vi "FTW-Actor-Broker-Initialize.vi"(0 "FTW Message Broker":refnum<class "FTW-Actor-Broker.lvclass">, 5 "Initialized Response":string, 11 "error in":errorcluster) -> (4 "FTW Message Broker out":refnum<class "FTW-Actor-Broker.lvclass">, 6 "Observer":refnum<event-registration>, 15 "error out":errorcluster)   [LabVIEW 2012, in "FTW-Actor-Broker.lvclass"]
uses:
  FTW-Actor-Broker.lvclass
  Messaging/Message/FTW-Message.lvclass
  Container/FTW-Container.lvclass
panel:
  # "Inputs"
  # "Outputs"
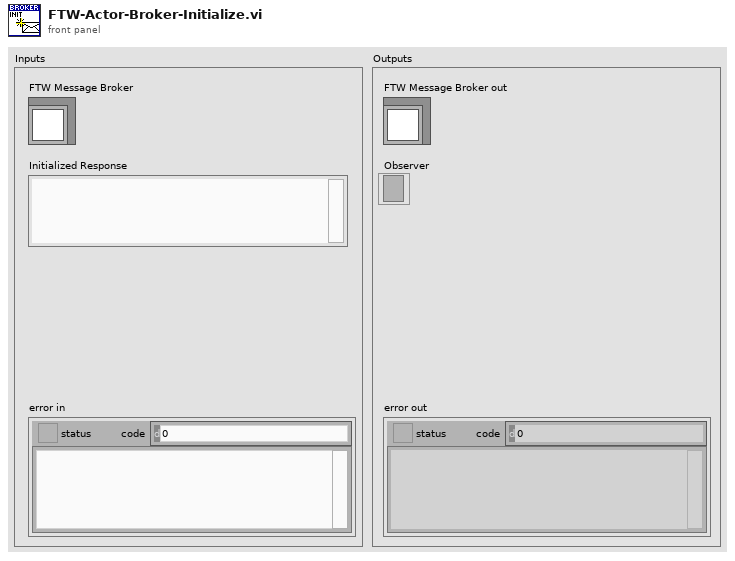
[diagram p1: front panel]
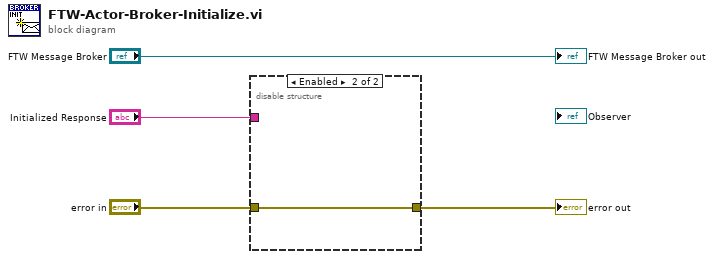
[diagram p0: block diagram]
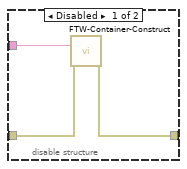
[diagram p2: hidden frame]
diagram:
  n1 = disable-structure shown="Enabled" {
    disable-tunnel: "Initialized Response" -> [w7 _]
    disable-tunnel: "error in" -> [w6 w8]
    disable-tunnel: [w5 w8] -> w1
    frame Disabled {
      n2 = call "FTW-Container-Construct.vi"("LabVIEW Data Structure"=w7, "error in"=w6) -> ("error out"=w5:errorcluster)  [unwired: 12 in, 1 out]
    }
    frame Enabled {
    }
  }
  "error out" <- w1
  "FTW Message Broker out" <- "FTW Message Broker"
